vi "6-2.vi"() -> ()   [LabVIEW 2019, in "6.lvlib"]
uses:
  6.lvlib
panel:
  out "N Lanternfish":i64
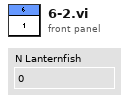
[diagram p1: front panel]
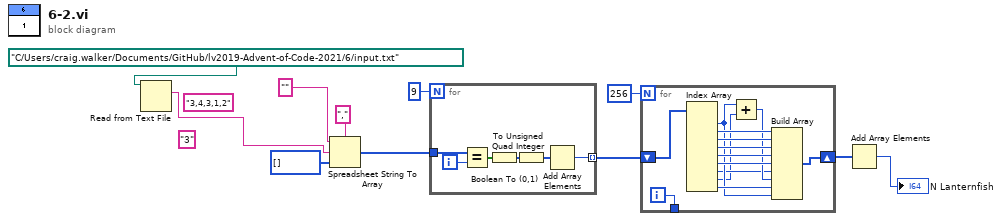
[diagram p0: block diagram]
diagram:
  (unwired) "3"
  (unwired) "3,4,3,1,2"
  n1 = Read from Text File(file (use dialog)=path "C:/Users/craig.walker/Documents/GitHub/lv2019-Advent-of-Code-2021/6/input.txt" ("file path (dialog if empty)")) -> (text=w1:string)  [unwired: 3 in, 3 out]
  n2 = Spreadsheet String To Array(delimiter (Tab)=",", format string="", spreadsheet string=w1, array type (2D Dbl)=u16[] []) -> (array=w6:u16[])
  n3 = for {
    N: 9 -> [_]
    tunnel: w6 -> [w17]
    tunnel: [w13] -> w5 mode=indexing
    i -> [w16]
    n4 = Equal?(x=w17, y=w16) -> (x = y?=w15:bool[])
    n5 = Boolean To (0,1)(Boolean=w15) -> (0, 1=w14:i16[])
    n6 = To Unsigned Quad Integer(1:w14) -> (0:w12:u64[])
    n7 = Add Array Elements(numeric array=w12) -> (sum=w13:u64)
  }
  n8 = for {
    N: 256 -> [_]
    shift-right: [w22] -> w3
    shift-left: w5 -> [w30]
    tunnel: [w21] -> _
    i -> [w21]
    n9 = Index Array(array=w30) -> (element #1=w23:u64, element #2=w29:u64, element #3=w28:u64, element #4=w27:u64, element #5=w26:u64, element #6=w25:u64, element #7=w19:u64, element #8=w18:u64, element #9=w24:u64)  [unwired: 9 in]
    n10 = Add(x=w23, y=w18) -> (x+y=w20:u64)
    n11 = Build Array(w29, w28, w27, w26, w25, w19, w20, w24, w23) -> (w22:u64[])
  }
  n12 = Add Array Elements(numeric array=w3) -> (sum=→"N Lanternfish":u64)
